vi "Play - Config File.vi"() -> ()   [LabVIEW 2020]
panel:
  in  "Quit":bool
  in  "Save":bool
  in  "Load":bool
  in  "Digital Meter":T1={"Type"="34401A", "VISA resource name"="GPIB0::17"}
  in  "String 1":string="Hello"
  in  "File Path":path=path "d:/temp.txt"
  in  "Value Integer":i32=63
  in  "Value Boolean":bool=TRUE
  in  "Value Floating":dbl=3.141
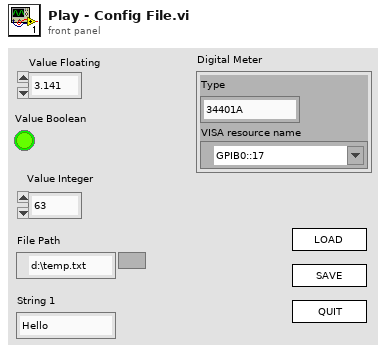
[diagram p1: front panel]
types:
  T1 = cluster{"Type":string, "VISA resource name":refnum<visa-resource-name>}
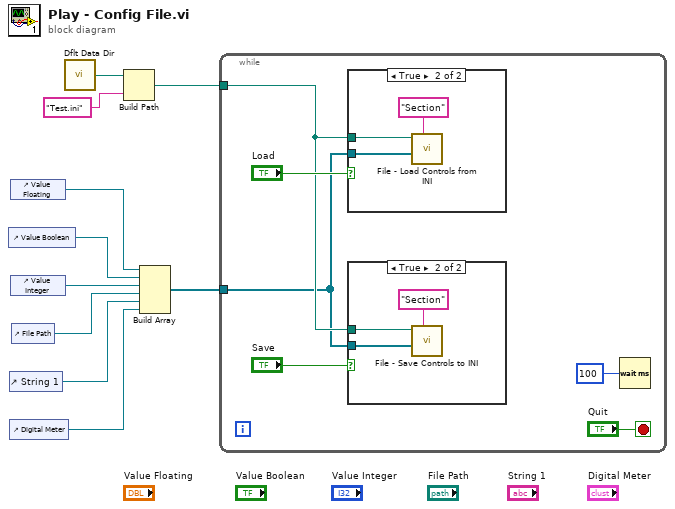
[diagram p0: block diagram]
diagram:
  n1 = control-ref of="Value Boolean"() -> (w6:refnum<vi>)
  n2 = control-ref of="String 1"() -> (w9:refnum<vi>)
  n3 = control-ref of="Digital Meter"() -> (w10:refnum<vi>)
  n4 = control-ref of="Value Floating"() -> (w5:refnum<vi>)
  n5 = control-ref of="Value Integer"() -> (w7:refnum<vi>)
  n6 = control-ref of="File Path"() -> (w8:refnum<vi>)
  n7 = call <vilib>:"Dflt Data Dir.vi"() -> ("App:Default Data Directory"=w3:path)
  n8 = Build Path(base path=w3, name or relative path="Test.ini") -> (appended path=w1:path)
  n9 = Build Array(w5, w6, w7, w8, w9, w10) -> (w4:refnum<vi>[])
  n10 = while {
    tunnel: w4 -> [w11]
    tunnel: w1 -> [w12]
    stop <- "Quit" stop-if-true
    n11 = case shown="True" "Load" {
      tunnel: w12 -> [_ w21]
      tunnel: w11 -> [_ w20]
      frame False {
      }
      frame True {
        n12 = call "File - Load Controls from INI.vi"("Section"="Section", "Array of References"=w20, "INI File"=w21) -> ()  [unwired: 8 in, 1 out]
      }
    }
    n13 = case shown="True" "Save" {
      tunnel: w12 -> [_ w18]
      tunnel: w11 -> [_ w17]
      frame False {
      }
      frame True {
        n14 = call "File - Save Controls to INI.vi"("Section"="Section", "Array of References"=w17, "INI File"=w18) -> ()  [unwired: 8 in, 1 out]
      }
    }
    n15 = Wait (ms)(milliseconds to wait=u32 100) -> ()  [unwired: 1 out]
  }
